vi "Day15-2.vi"() -> ()   [LabVIEW 2021]
panel:
  out "tuning f":u64
  out "XY Graph":cluster{i32[], i32[]}[](graph)
  out "Array 9":i32[](array[numeric])
  out "Array 7":string[](array[string])
  out "sum 2":i32
  out "sum":i32
  out "Array 6":string[][](array[string])
  out "Array 5":string[][](array[string])
  out "min y":i32
  out "max y":i32
  out "min x":i32
  out "max x":i32
  out "Array 4":i32[](array[numeric])
  out "beacons":cluster{i32, i32}[](array[cluster])
  out "sensprs":cluster{i32, i32}[](array[cluster])
  out "sensors":i32
  out "Array":string[](array[string])
  out "array":string[][](array[string])
  # "5917380"
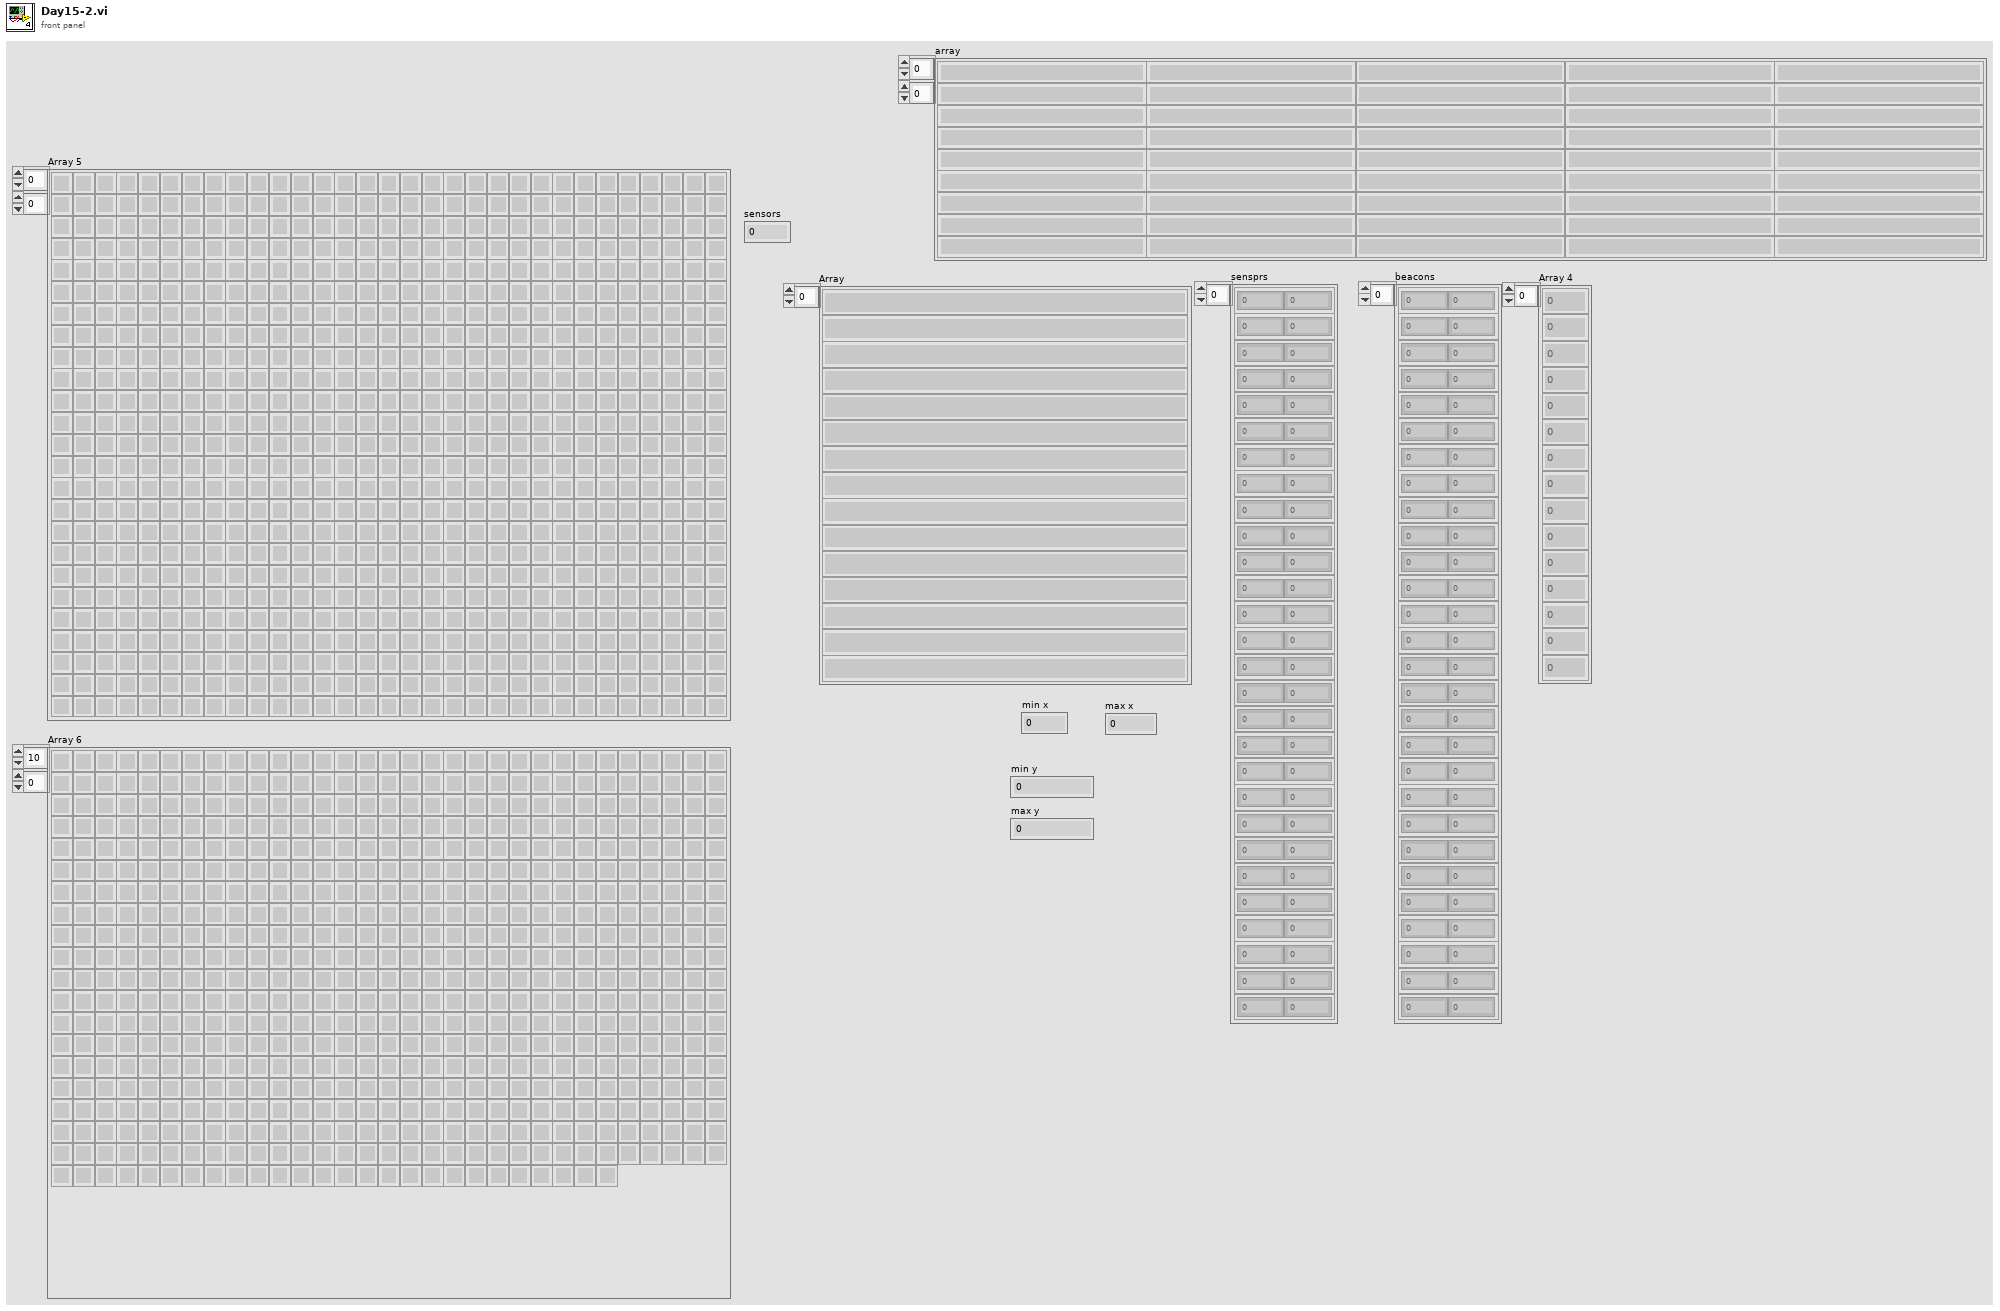
[diagram p1: front panel]
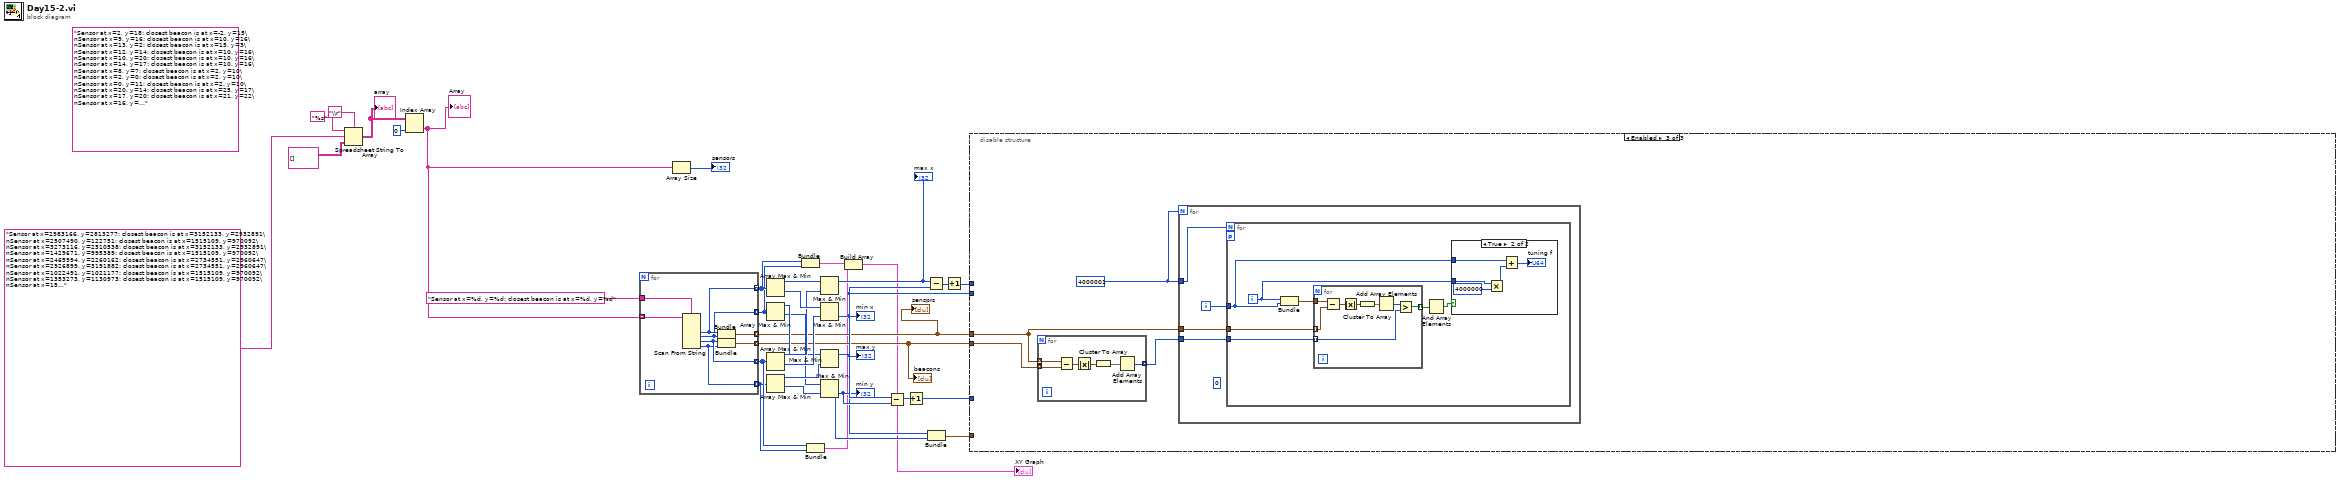
[diagram p0: block diagram]
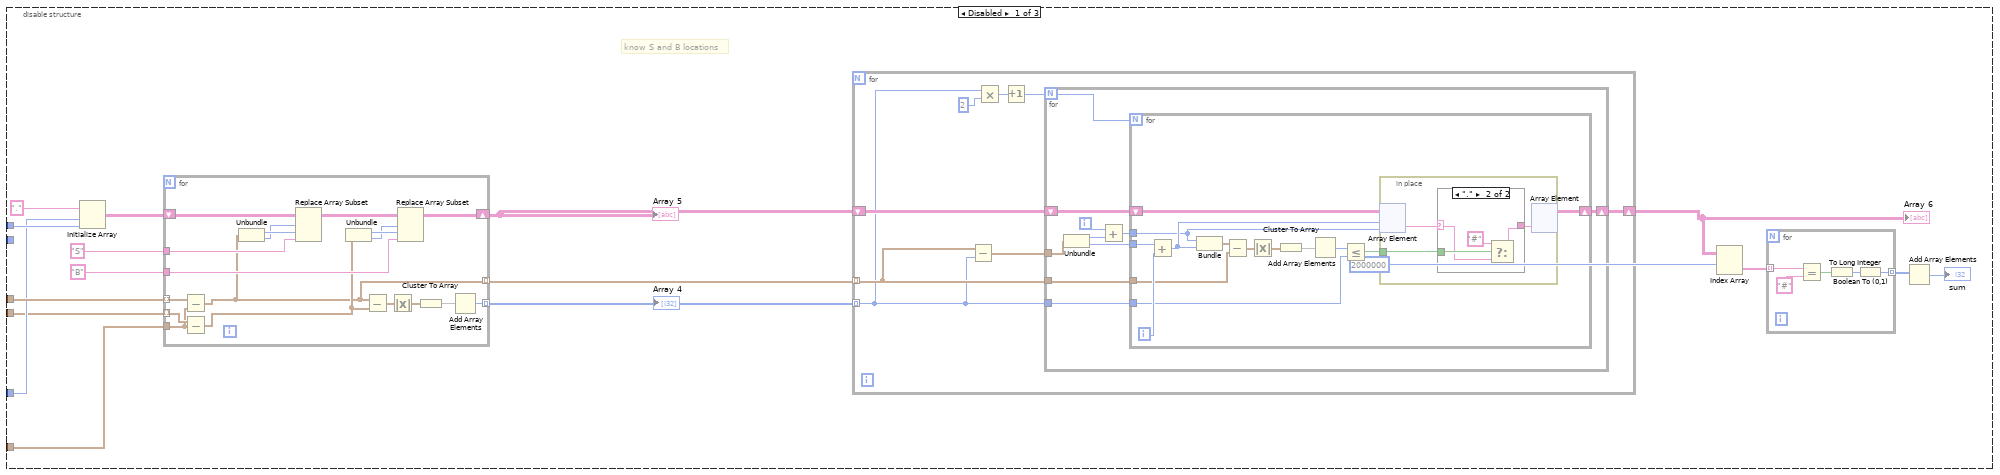
[diagram p2: hidden frame]
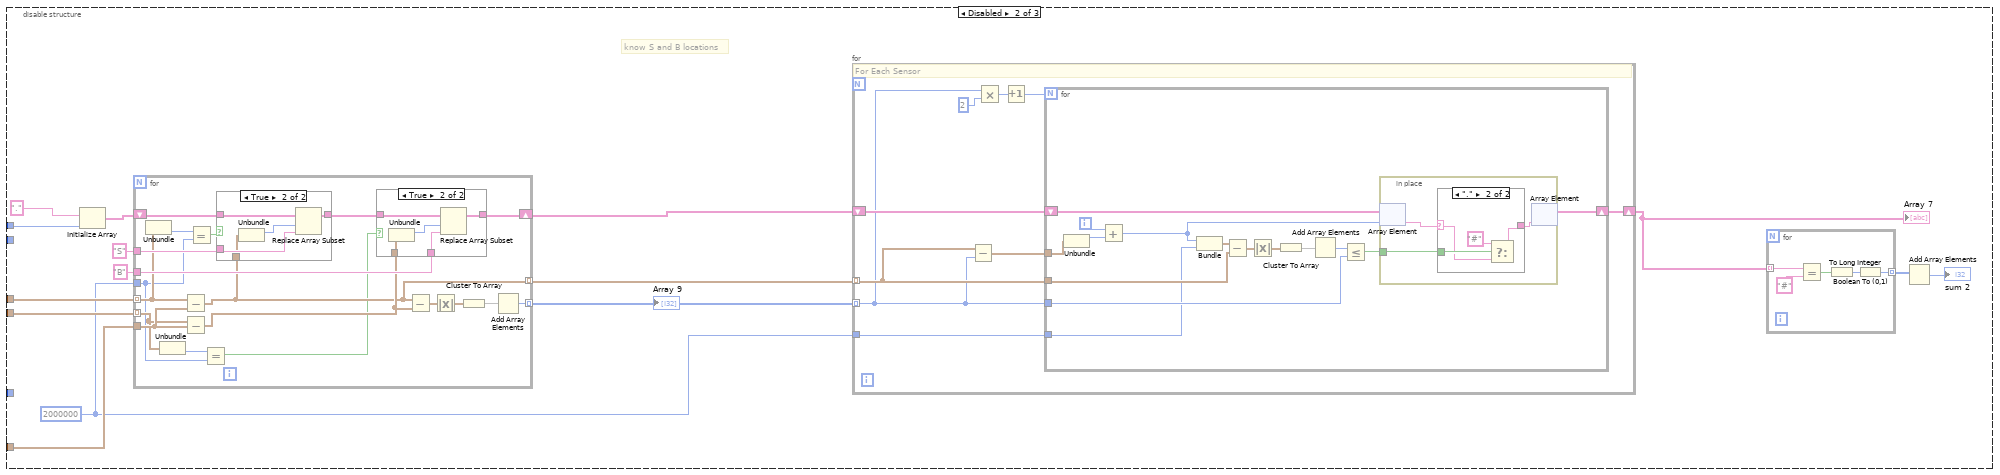
[diagram p4: hidden frame]
diagram:
  (unwired) "Sensor at x=2, y=18: closest beacon is at x=-2, y=15\nSensor at x=9, y=16: closest beacon is at x=10, y=16\nSensor at x=13, y=2: closest beacon is at x=15, y=3\nSensor at x=12, y=14: closest beacon is at x=10, y=16\nSensor at x=10, y=20: closest beacon is at x=10, y=16\nSensor at x=14, y=17: closest beacon is at x=10, y=16\nSensor at x=8, y=7: closest beacon is at x=2, y=10\nSensor at x=2, y=0: closest beacon is at x=2, y=10\nSensor at x=0, y=11: closest beacon is at x=2, y=10\nSensor at x=20, y=14: closest beacon is at x=25, y=17\nSensor at x=17, y=20: closest beacon is at x=21, y=22\nSensor at x=16, y=7: closest beacon is at x=15, y=3\nSensor at x=14, y=3: closest beacon is at x=15, y=3\nSensor at x=20, y=1: closest beacon is at x=15, y=3"
  n1 = Spreadsheet String To Array(delimiter (Tab)="\\r", format string="%s", spreadsheet string="Sensor at x=2983166, y=2813277: closest beacon is at x=3152133, y=2932891\nSensor at x=2507490, y=122751: closest beacon is at x=1515109, y=970092\nSensor at x=3273116, y=2510538: closest beacon is at x=3152133, y=2932891\nSensor at x=1429671, y=995389: closest beacon is at x=1515109, y=970092\nSensor at x=2465994, y=2260162: closest beacon is at x=2734551, y=2960647\nSensor at x=2926899, y=3191882: closest beacon is at x=2734551, y=2960647\nSensor at x=1022491, y=1021177: closest beacon is at x=1515109, y=970092\nSensor at x=1353273, y=1130973: closest beacon is at x=1515109, y=970092\nSensor at x=1565476, y=2081049: closest beacon is at x=1597979, y=2000000\nSensor at x=1841125, y=1893566: closest beacon is at x=1597979, y=2000000\nSensor at x=99988, y=71317: closest beacon is at x=86583, y=-1649857\nSensor at x=3080600, y=3984582: closest beacon is at x=3175561, y=4138060\nSensor at x=3942770, y=3002123: closest beacon is at x=3724687, y=3294321\nSensor at x=1572920, y=2031447: closest beacon is at x=1597979, y=2000000\nSensor at x=218329, y=1882777: closest beacon is at x=1597979, y=2000000\nSensor at x=1401723, y=1460526: closest beacon is at x=1515109, y=970092\nSensor at x=2114094, y=985978: closest beacon is at x=1515109, y=970092\nSensor at x=3358586, y=3171857: closest beacon is at x=3152133, y=2932891\nSensor at x=1226284, y=3662922: closest beacon is at x=2514367, y=3218259\nSensor at x=3486366, y=3717867: closest beacon is at x=3724687, y=3294321\nSensor at x=1271873, y=831354: closest beacon is at x=1515109, y=970092\nSensor at x=3568311, y=1566400: closest beacon is at x=3152133, y=2932891\nSensor at x=3831960, y=3146611: closest beacon is at x=3724687, y=3294321\nSensor at x=2505534, y=3196726: closest beacon is at x=2514367, y=3218259\nSensor at x=2736967, y=3632098: closest beacon is at x=2514367, y=3218259\nSensor at x=3963402, y=3944423: closest beacon is at x=3724687, y=3294321\nSensor at x=1483115, y=2119639: closest beacon is at x=1597979, y=2000000", array type (2D Dbl)=string[][] []) -> (array=w31:string[][])
  "array" <- w31
  n2 = Index Array(array=w31, index (col)=0 ("disabled index (col)")) -> (element=w29:string[])  [unwired: 1 in]
  "Array" <- w29
  n3 = for {
    tunnel: w29 -> [w43] mode=indexing
    tunnel: "Sensor at x=%d, y=%d: closest beacon is at x=%d, y=%d" ("format string") -> [w42]
    tunnel: [w41] -> w8 mode=indexing
    tunnel: [w40] -> w9 mode=indexing
    tunnel: [w39] -> w5 mode=indexing
    tunnel: [w38] -> w4 mode=indexing
    tunnel: [w37] -> w7 mode=indexing
    tunnel: [w36] -> w6 mode=indexing
    n4 = Scan From String(format string=w42, input string=w43) -> (output 1=w39:i32, output 2=w38:i32, output 3=w37:i32, output 4=w36:i32)  [unwired: 6 in, 3 out]
    n5 = Bundle(w39, w38) -> (w41:cluster{i32, i32})  [unwired: 1 in]
    n6 = Bundle(w37, w36) -> (w40:cluster{i32, i32})  [unwired: 1 in]
  }
  "sensprs" <- w8
  "beacons" <- w9
  n7 = Array Size(array=w29) -> (size(s)=→"sensors":i32)
  n8 = Array Max & Min(array=w5) -> (max value=w27:i32, min value=w26:i32)  [unwired: 2 out]
  n9 = Array Max & Min(array=w4) -> (max value=w23:i32, min value=w20:i32)  [unwired: 2 out]
  n10 = Array Max & Min(array=w7) -> (max value=w25:i32, min value=w24:i32)  [unwired: 2 out]
  n11 = Array Max & Min(array=w6) -> (max value=w22:i32, min value=w21:i32)  [unwired: 2 out]
  n12 = Bundle(w5, w4) -> (w3:cluster{i32[], i32[]})  [unwired: 1 in]
  n13 = Bundle(w7, w6) -> (w2:cluster{i32[], i32[]})  [unwired: 1 in]
  n14 = Max & Min(x=w27, y=w25) -> (max(x,y)=w16:i32)  [unwired: 1 out]
  "max x" <- w16
  n15 = Max & Min(x=w26, y=w24) -> (min(x,y)=w11:i32)  [unwired: 1 out]
  "min x" <- w11
  n16 = Max & Min(x=w23, y=w22) -> (max(x,y)=w19:i32)  [unwired: 1 out]
  "max y" <- w19
  n17 = Max & Min(x=w20, y=w21) -> (min(x,y)=w13:i32)  [unwired: 1 out]
  "min y" <- w13
  n18 = Build Array(w3, w2) -> (→"XY Graph":cluster{i32[], i32[]}[])
  n19 = Subtract(x=w19, y=w13) -> (x-y=w18:i32)
  n20 = Increment(x=w18) -> (x+1=w14:i32)
  n21 = Subtract(x=w16, y=w11) -> (x-y=w17:i32)
  n22 = Bundle(w11, w13) -> (w12:cluster{i32, i32})  [unwired: 1 in]
  n23 = Increment(x=w17) -> (x+1=w15:i32)
  n24 = disable-structure shown="Enabled" {
    disable-tunnel: w8 -> [w60 w138 w209]
    disable-tunnel: w15 -> [w59 w137 _]
    disable-tunnel: w14 -> [w58 _ _]
    disable-tunnel: w9 -> [w56 w135 w210]
    disable-tunnel: w12 -> [w44 w125 _]
    disable-tunnel: w11 -> [_ _ _]
    frame Disabled {
      # "know S and B locations"
      n25 = Initialize Array("." ("x+1"), w58, w59) -> (w55:string[][])
      n26 = for {
        tunnel: w60 -> [w112] mode=indexing
        tunnel: w56 -> [w114] mode=indexing
        tunnel: [w120] -> w51 mode=indexing
        shift-right: [w115] -> w52
        shift-left: w55 -> [w119]
        tunnel: "B" ("x+1") -> [w116]
        tunnel: "S" ("x+1") -> [w118]
        tunnel: w44 -> [w113]
        tunnel: [w106] -> w50 mode=indexing
        n27 = Subtract(x=w112, y=w113) -> (x-y=w106:cluster{i32, i32})
        n28 = Subtract(x=w114, y=w113) -> (x-y=w107:cluster{i32, i32})
        n29 = Unbundle(w106) -> (w111:i32, w110:i32)
        n30 = Replace Array Subset(array=w119, new element=w118, index (row)=w110, index (col)=w111) -> (w117:string[][])
        n31 = Unbundle(w107) -> (w109:i32, w108:i32)
        n32 = Subtract(x=w106, y=w107) -> (x-y=w123:cluster{i32, i32})
        n33 = Absolute Value(x=w123) -> (abs(x)=w122:cluster{i32, i32})
        n34 = Replace Array Subset(array=w117, new element=w116, index (row)=w108, index (col)=w109) -> (w115:string[][])
        n35 = Cluster To Array(cluster=w122) -> (array=w121:i32[])
        n36 = Add Array Elements(numeric array=w121) -> (sum=w120:i32)
      }
      "Array 4" <- w51
      "Array 5" <- w52
      n37 = for {
        shift-right: [w72] -> w48
        shift-left: w52 -> [w73]
        tunnel: w51 -> [w67] mode=indexing
        tunnel: w50 -> [w68] mode=indexing
        n38 = Subtract(x=w68, y=w67) -> (x-y=w66:cluster{i32, i32})
        n39 = Multiply(x=w67, y=2) -> (x*y=w70:i32)
        n40 = Increment(x=w70) -> (x+1=w69:i32)
        n41 = for {
          N: w69 -> [w79]
          shift-right: [w80] -> w72
          shift-left: w73 -> [w83]
          tunnel: w68 -> [w82]
          tunnel: w67 -> [w81]
          tunnel: w66 -> [w78]
          i -> [w76]
          n42 = Unbundle(w78) -> (w77:i32, w75:i32)
          n43 = Add(x=w76, y=w77) -> (x+y=w74:i32)
          n44 = for {
            N: w79 -> [_]
            shift-right: [w84] -> w80
            shift-left: w83 -> [w88]
            tunnel: w82 -> [w92]
            tunnel: w81 -> [w89]
            tunnel: w75 -> [w97]
            tunnel: w74 -> [w86]
            i -> [w96]
            n45 = Add(x=w97, y=w96) -> (x+y=w87:i32)
            n46 = Bundle(w86, w87) -> (w91:cluster{i32, i32})  [unwired: 1 in]
            n47 = Subtract(x=w91, y=w92) -> (x-y=w95:cluster{i32, i32})
            n48 = Absolute Value(x=w95) -> (abs(x)=w94:cluster{i32, i32})
            n49 = Cluster To Array(cluster=w94) -> (array=w93:i32[])
            n50 = Add Array Elements(numeric array=w93) -> (sum=w90:i32)
            n51 = Less Or Equal?(x=w90, y=w89) -> (x <= y?=w85:bool)
            n52 = in-place {
              in-place-border: w85 -> [w98]
              n53 = in-place-array #1(w88, w87, w86) -> (w100:string)
              n54 = case shown="\".\"" w100 {
                selector: w100 -> [w101 w104]
                tunnel: [w101 w102] -> w99
                tunnel: w98 -> [_ w105]
                frame Default {
                }
                frame "." {
                  n55 = Select(t="#" ("x+1"), s=w105, f=w104) -> (s? t:f=w102:string)
                }
              }
              n56 = in-place-array #1(w99) -> (w84:string[][])  [unwired: 2 out]
            }
          }
        }
      }
      "Array 6" <- w48
      n57 = Index Array(array=w48, index (row)=2000000) -> (element=w47:string[])  [unwired: 1 in]
      n58 = for {
        tunnel: w47 -> [w65] mode=indexing
        tunnel: [w61] -> w46 mode=indexing
        n59 = Equal?(x=w65, y="#" ("x+1")) -> (x = y?=w63:bool)
        n60 = Boolean To (0,1)(Boolean=w63) -> (0, 1=w62:i16)
        n61 = To Long Integer(number=w62) -> (32bit integer=w61:i32)
      }
      n62 = Add Array Elements(numeric array=w46) -> (sum=→"sum":i32)
    }
    frame Disabled {
      w124 = 2000000 ("index (row)")
      # "know S and B locations"
      n63 = Initialize Array("." ("x+1"), w137) -> (w134:string[])
      n64 = for {
        tunnel: w138 -> [w182] mode=indexing
        tunnel: w135 -> [w178] mode=indexing
        tunnel: [w191] -> w130 mode=indexing
        shift-right: [w186] -> w131
        shift-left: w134 -> [w190]
        tunnel: "B" ("x+1") -> [w187]
        tunnel: "S" ("x+1") -> [w189]
        tunnel: w125 -> [w185]
        tunnel: [w183] -> w129 mode=indexing
        tunnel: w124 -> [w177]
        n65 = Unbundle(w182) -> (w181:i32)  [unwired: 1 out]
        n66 = Unbundle(w178) -> (w179:i32)  [unwired: 1 out]
        n67 = Subtract(x=w182, y=w185) -> (x-y=w183:cluster{i32, i32})
        n68 = Subtract(x=w178, y=w185) -> (x-y=w184:cluster{i32, i32})
        n69 = Equal?(x=w181, y=w177) -> (x = y?=w180:bool)
        n70 = Equal?(x=w179, y=w177) -> (x = y?=w176:bool)
        n71 = case shown="True" w180 {
          tunnel: w190 -> [w201 w206]
          tunnel: w189 -> [_ w205]
          tunnel: [w201 w204] -> w188
          tunnel: w183 -> [_ w203]
          frame False {
          }
          frame True {
            n72 = Unbundle(w203) -> (w202:i32)  [unwired: 1 out]
            n73 = Replace Array Subset(array=w206, new element=w205, index=w202) -> (w204:string[])
          }
        }
        n74 = case shown="True" w176 {
          tunnel: w188 -> [w195 w200]
          tunnel: w187 -> [_ w199]
          tunnel: [w195 w198] -> w186
          tunnel: w184 -> [_ w197]
          frame False {
          }
          frame True {
            n75 = Unbundle(w197) -> (w196:i32)  [unwired: 1 out]
            n76 = Replace Array Subset(array=w200, new element=w199, index=w196) -> (w198:string[])
          }
        }
        n77 = Subtract(x=w183, y=w184) -> (x-y=w194:cluster{i32, i32})
        n78 = Absolute Value(x=w194) -> (abs(x)=w193:cluster{i32, i32})
        n79 = Cluster To Array(cluster=w193) -> (array=w192:i32[])
        n80 = Add Array Elements(numeric array=w192) -> (sum=w191:i32)
      }
      "Array 9" <- w130
      n81 = for {
        shift-right: [w151] -> w128
        shift-left: w131 -> [w152]
        tunnel: w130 -> [w146] mode=indexing
        tunnel: w129 -> [w147] mode=indexing
        tunnel: w124 -> [w144]
        # "For Each Sensor"
        n82 = Subtract(x=w147, y=w146) -> (x-y=w145:cluster{i32, i32})
        n83 = Multiply(x=w146, y=2) -> (x*y=w149:i32)
        n84 = Increment(x=w149) -> (x+1=w148:i32)
        n85 = for {
          N: w148 -> [_]
          shift-right: [w164] -> w151
          shift-left: w152 -> [w167]
          tunnel: w147 -> [w166]
          tunnel: w146 -> [w165]
          tunnel: w145 -> [w163]
          tunnel: w144 -> [w153]
          i -> [w161]
          n86 = Unbundle(w163) -> (w162:i32)  [unwired: 1 out]
          n87 = Add(x=w161, y=w162) -> (x+y=w154:i32)
          n88 = Bundle(w154, "index (row)"=w153) -> (w157:cluster{i32, "index (row)":i32})  [unwired: 1 in]
          n89 = Subtract(x=w157, y=w166) -> (x-y=w160:cluster{i32, i32})
          n90 = Absolute Value(x=w160) -> (abs(x)=w159:cluster{i32, i32})
          n91 = Cluster To Array(cluster=w159) -> (array=w158:i32[])
          n92 = Add Array Elements(numeric array=w158) -> (sum=w156:i32)
          n93 = Less Or Equal?(x=w156, y=w165) -> (x <= y?=w155:bool)
          n94 = in-place {
            in-place-border: w155 -> [w168]
            n95 = in-place-array #2(w167, w154) -> (w170:string)
            n96 = case shown="\".\"" w170 {
              selector: w170 -> [w171 w174]
              tunnel: [w171 w172] -> w169
              tunnel: w168 -> [_ w175]
              frame Default {
              }
              frame "." {
                n97 = Select(t="#" ("x+1"), s=w175, f=w174) -> (s? t:f=w172:string)
              }
            }
            n98 = in-place-array #2(w169) -> (w164:string[])  [unwired: 1 out]
          }
        }
      }
      "Array 7" <- w128
      n99 = for {
        tunnel: w128 -> [w143] mode=indexing
        tunnel: [w139] -> w127 mode=indexing
        n100 = Equal?(x=w143, y="#" ("x+1")) -> (x = y?=w141:bool)
        n101 = Boolean To (0,1)(Boolean=w141) -> (0, 1=w140:i16)
        n102 = To Long Integer(number=w140) -> (32bit integer=w139:i32)
      }
      n103 = Add Array Elements(numeric array=w127) -> (sum=→"sum 2":i32)
    }
    frame Enabled {
      w207 = 4000001
      n104 = for {
        tunnel: w209 -> [w237] mode=indexing
        tunnel: w210 -> [w236] mode=indexing
        tunnel: [w235] -> w208 mode=indexing
        n105 = Subtract(x=w237, y=w236) -> (x-y=w240:cluster{i32, i32})
        n106 = Absolute Value(x=w240) -> (abs(x)=w239:cluster{i32, i32})
        n107 = Cluster To Array(cluster=w239) -> (array=w238:i32[])
        n108 = Add Array Elements(numeric array=w238) -> (sum=w235:i32)
      }
      n109 = for {
        N: w207 -> [_]
        tunnel: w209 -> [w214]
        tunnel: w208 -> [w213]
        tunnel: w207 -> [w212]
        i -> [w211]
        (unwired) 0
        n110 = for {
          N: w212 -> [_]
          tunnel: w211 -> [w216]
          tunnel: w214 -> [w220]
          tunnel: w213 -> [w219]
          workers-P: _ -> [_]
          i -> [w217]
          n111 = Bundle(w217, w216) -> (w221:cluster{i32, i32})  [unwired: 1 in]
          n112 = for {
            tunnel: w221 -> [w231]
            tunnel: w220 -> [w230] mode=indexing
            tunnel: w219 -> [w228] mode=indexing
            tunnel: [w227] -> w218 mode=indexing
            n113 = Subtract(x=w231, y=w230) -> (x-y=w232:cluster{i32, i32})
            n114 = Absolute Value(x=w232) -> (abs(x)=w233:cluster{i32, i32})
            n115 = Cluster To Array(cluster=w233) -> (array=w234:i32[])
            n116 = Add Array Elements(numeric array=w234) -> (sum=w229:i32)
            n117 = Greater?(x=w229, y=w228) -> (0:w227:bool)
          }
          n118 = And Array Elements(Boolean array=w218) -> (logical AND=w215:bool)
          n119 = case shown="True" w215 {
            tunnel: w217 -> [_ w223]
            tunnel: w216 -> [_ w222]
            frame False {
            }
            frame True {
              n120 = Multiply(x=w223, y=u64 4000000) -> (x*y=w225:u64)
              n121 = Add(x=w222, y=w225) -> (x+y=→"tuning f":u64)
            }
          }
        }
      }
    }
  }
